vi "shared Variable as Variant Test.vi"() -> ()   [LabVIEW 2021]
uses:
  Source/Omni-Bus/Omni_Bus.lvclass
  Source/Local Vars/Local Vars.lvclass
  Source/Omni-Bus/Support/Broad Types.ctl
  <vilib>/TSA/LVabs_Shared Variable/Bool/conc_SharedVar_Bool.lvclass
  <vilib>/TSA/LVabs_Shared Variable/DBL/conc_SharedVar_DBL.lvclass
  <vilib>/TSA/Abstract Data Classes/Abs_Types/Boolean/Static Write.vi
  <vilib>/TSA/Abstract Data Classes/Abs_Types/Boolean/Abs_Boolean.lvclass
  <vilib>/TSA/Abstract Data Classes/Abs_Types/Double Float/Static Write.vi
  <vilib>/TSA/Abstract Data Classes/Abs_Types/Double Float/Abs_Double Float.lvclass
  C:/Program Files (x86)/National Instruments/LabVIEW 2021/vi.lib/TSA/Abstract Data Classes/Abs_Types/Boolean/Abs_Boolean.lvclass
  C:/Program Files (x86)/National Instruments/LabVIEW 2021/vi.lib/TSA/Abstract Data Classes/Abs_Types/Value/Abs_Value.lvclass
  C:/Program Files (x86)/National Instruments/LabVIEW 2021/vi.lib/TSA/Abstract Data Classes/Abs_Types/Type/Abs_Type.lvclass
  C:/Program Files (x86)/National Instruments/LabVIEW 2021/vi.lib/TSA/LVabs_Shared Variable/Bool/conc_SharedVar_Bool.lvclass
  C:/Program Files (x86)/National Instruments/LabVIEW 2021/vi.lib/TSA/LVabs_Shared Variable/Interface/abs_SharedVariable.lvclass
  C:/Program Files (x86)/National Instruments/LabVIEW 2021/vi.lib/TSA/Abstract Data Classes/Abs_Types/Double Float/Abs_Double Float.lvclass
  C:/Program Files (x86)/National Instruments/LabVIEW 2021/vi.lib/TSA/Abstract Data Classes/Abs_Types/Floating Point/Abs_Floating Point.lvclass
  C:/Program Files (x86)/National Instruments/LabVIEW 2021/vi.lib/TSA/Abstract Data Classes/Abs_Types/Numeric/Abs_Numeric.lvclass
  C:/Program Files (x86)/National Instruments/LabVIEW 2021/vi.lib/TSA/LVabs_Shared Variable/DBL/conc_SharedVar_DBL.lvclass
  <vilib>/TSA/Abstract Data Classes/Abs_Types/Value/Abs_Value.lvclass
  C:/Users/Tim/Documents/GitHub/Omni-Bus/Source/Bus_Access/Bus_Access.lvclass
  C:/Users/Tim/Documents/GitHub/Omni-Bus/Source/Local Vars/Local Vars.lvclass
  <vilib>/TSA/Abstract Data Classes/Abs_Types/Double Float/Support/Type.ctl
panel:
  in  "Boolean":bool
  out "error out 2":errorcluster
  out "error out":errorcluster
  in  "Tag 2":string
  in  "Tag":string
  out "Variant":variant
  in  "Value 2":T1
  in  "stop 2":bool
  in  "stop":bool
  out "Tags":string[](array[string])
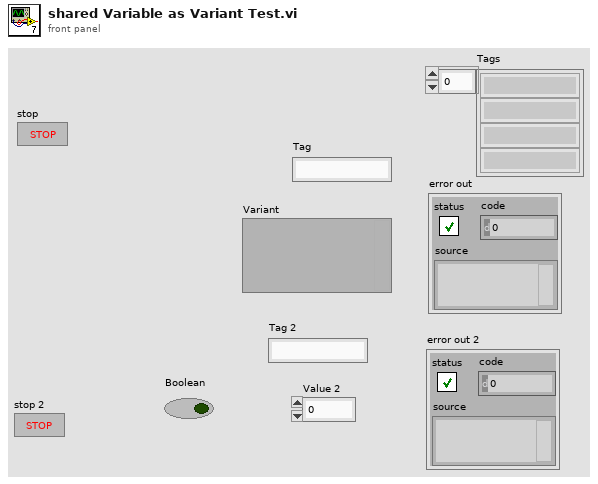
[diagram p1: front panel]
types:
  T1 = typedef "Abs_Double Float.lvclass/Type.ctl" = dbl
  T2 = typedef "Omni_Bus.lvclass/Broad Types.ctl" = enum16{"All Tags", "NI Specific Type", "Boolean", "String", "Numeric", "Float", "Integer", "Collection", "All Value Types", "Non Value Types"}
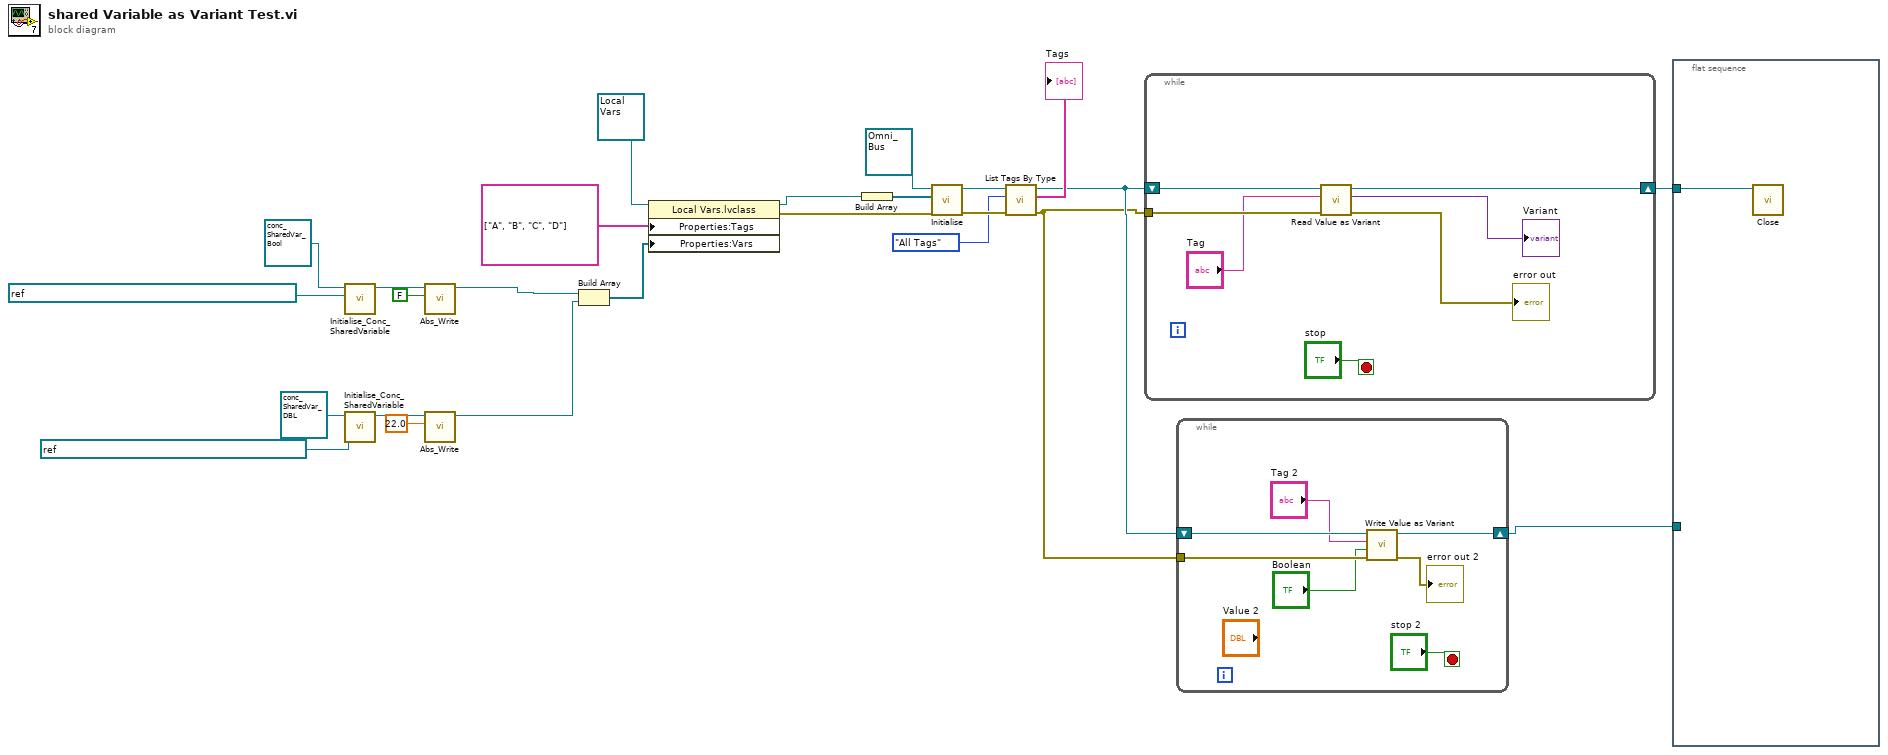
[diagram p0: block diagram]
diagram:
  n1 = call-poly <vilib>:"Initialise_Conc_SharedVariable.vi"("shared variable refnum"=refnum<k21> "ni.var.psp://my computer/Test Variables/Boolean", "abs_SharedVar_Bool in"=refnum<class "conc_SharedVar_Bool.lvclass"> refnum) -> ("abs_SharedVar_Bool out"=w6:refnum<class "conc_SharedVar_Bool.lvclass">)  [unwired: 8 in, 1 out]
  n2 = call-poly <vilib>:"Initialise_Conc_SharedVariable.vi"("shared variable refnum"=refnum<k21> "ni.var.psp://my computer/Test Variables/DBL", "abs_SharedVar_Bool in"=refnum<class "conc_SharedVar_DBL.lvclass"> refnum) -> ("abs_SharedVar_Bool out"=w3:refnum<class "conc_SharedVar_DBL.lvclass">)  [unwired: 8 in, 1 out]
  n3 = call-poly <vilib>:"Abs_Write.vi"("Boolean"=FALSE, "Abs_Boolean in"=w6) -> ("Abs_Boolean out"=w5:refnum<class "conc_SharedVar_Bool.lvclass">)  [unwired: 8 in, 1 out]
  n4 = call-poly <vilib>:"Abs_Write.vi"("Value"=22.0, "Abs_Double Float in"=w3) -> ("Abs_Double Float out"=w1:refnum<class "conc_SharedVar_DBL.lvclass">)  [unwired: 8 in, 1 out]
  n5 = Build Array(w5, w1) -> (w19:refnum<class "Abs_Value.lvclass">[])
  n6 = property class="Local Vars.lvclass"(reference=refnum<class "Local Vars.lvclass"> refnum ("Data in"), "Properties:Tags"=string[] ["A", "B", "C", "D"] ("Tags"), "Properties:Vars"=w19) -> (reference out=w22:refnum<class "Local Vars.lvclass">, error out=w23:errorcluster)  [unwired: 1 in]
  n7 = Build Array(w22) -> (w24:refnum<class "Local Vars.lvclass">[])
  n8 = call-dynamic <vilib>:"Initialise.vi"("error in (no error)"=w23, "Var Access"=w24, "Var Bus in"=refnum<class "Omni_Bus.lvclass"> refnum) -> ("error out"=w17:errorcluster, "Var Bus out"=w18:refnum<class "Omni_Bus.lvclass">)  [unwired: 7 in]
  n9 = call-dynamic "List Tags By Type.vi"("error in (no error)"=w17, "Broad Types"=Broad_Types."All Tags", "Var Bus in"=w18) -> ("error out"=w12:errorcluster, "Tags"=→"Tags":string[], "Var Bus out"=w13:refnum<class "Omni_Bus.lvclass">)  [unwired: 5 in, 1 out]
  n10 = while {
    shift-right: [w28] -> w14
    shift-left: w13 -> [w29]
    tunnel: w12 -> [w31]
    stop <- "stop" stop-if-true
    n11 = call "Read Value as Variant.vi"("error in (no error)"=w31, "Tag"="Tag", "Var Bus in"=w29) -> ("error out"=→"error out":errorcluster, "Variant"=→"Variant":variant, "Var Bus out"=w28:refnum<class "Omni_Bus.lvclass">)  [unwired: 6 in]
  }
  n12 = while {
    shift-right: [w37] -> w7
    shift-left: w13 -> [w38]
    tunnel: w12 -> [w36]
    stop <- "stop 2" stop-if-true
    n13 = call "Write Value as Variant.vi"("error in (no error)"=w36, "Variant"="Boolean", "Tag"="Tag 2", "Var Bus in"=w38) -> ("error out"=→"error out 2":errorcluster, "Var Bus out"=w37:refnum<class "Omni_Bus.lvclass">)  [unwired: 6 in]
  }
  n14 = flat-sequence {
    tunnel: w14 -> [w40]
    tunnel: w7 -> [_]
    frame #0 {
      n15 = call-dynamic "Close.vi"("Data in"=w40) -> ()  [unwired: 9 in, 2 out]
    }
  }
